vi "MSGR subVI_template 2.vi"(8 "error in (no error)":errorcluster, 11 "MSGR Q name":T1) -> (0 "error out":errorcluster)   [LabVIEW 2018]
uses:
  MSGR Q Name TypeDef.ctl
  MSGR Send (Name).vi
  MSGR Get Q.vi
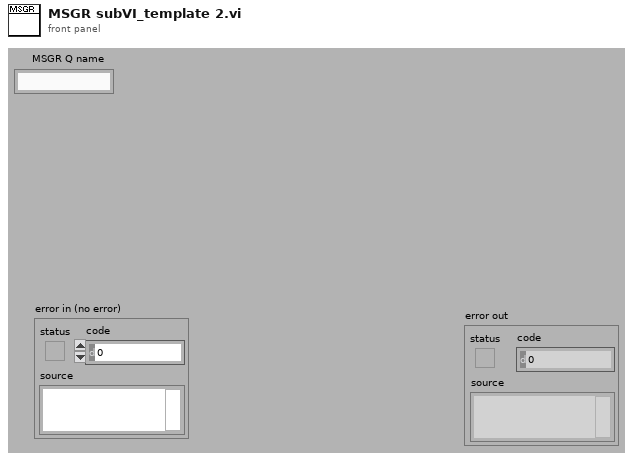
[diagram p1: front panel]
types:
  T1 = typedef "MSGR Q Name TypeDef.ctl" = string
  T2 = typedef "MSGR Q Data TypeDef.ctl" = cluster{"Msg":string, "Parameters":string, "Reply?":bool, "ReplyQ":string}
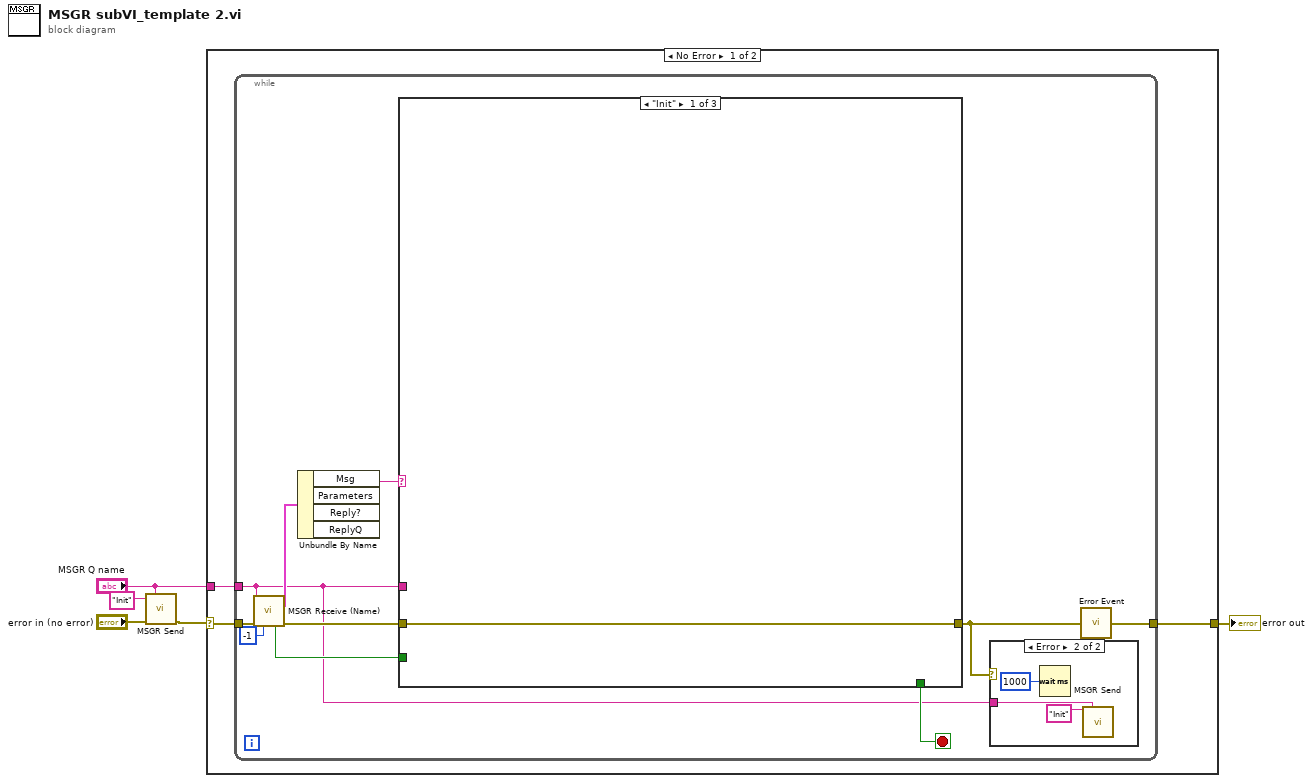
[diagram p0: block diagram]
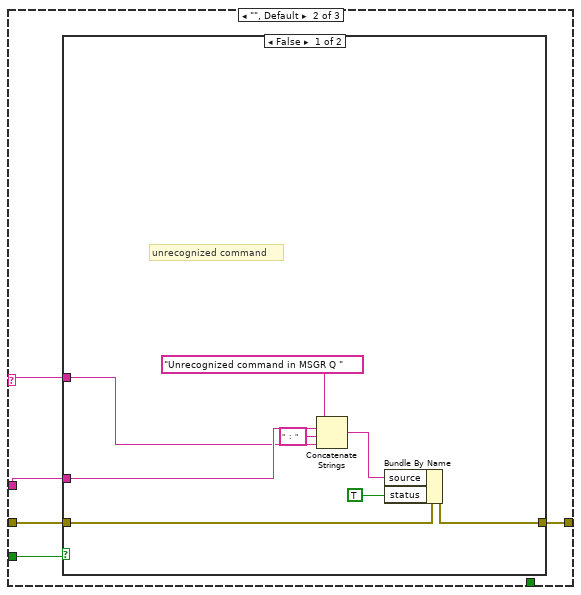
[diagram p3: hidden frame]
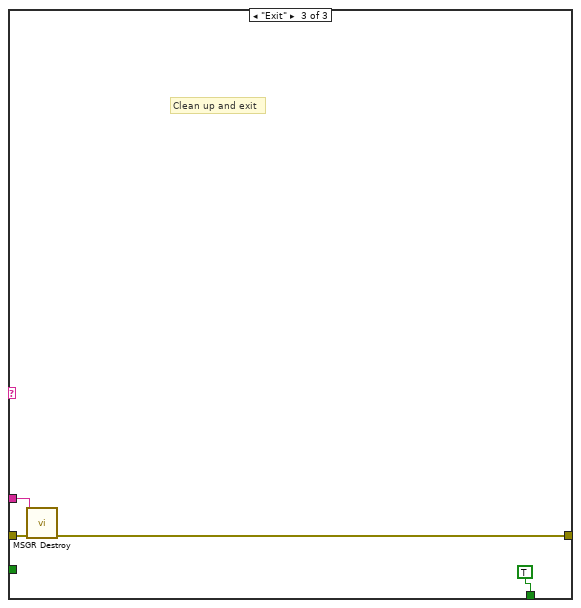
[diagram p5: hidden frame]
diagram:
  n1 = call-poly "MSGR Send.vi"("Msg"="Init", "MSGR Q name"="MSGR Q name", "error in (no error)"="error in (no error)") -> ("error out"=w4:errorcluster)  [unwired: 11 in, 1 out]
  n2 = case shown="No Error" w4 {
    selector: w4 -> [w8 w41]
    tunnel: [w7 w41] -> w5
    tunnel: "MSGR Q name" -> [w6 _]
    frame No Error {
      n3 = while {
        tunnel: w8 -> [w18]
        tunnel: [w11] -> w7
        tunnel: w6 -> [w9]
        stop <- w14 stop-if-true
        n4 = call "MSGR Receive (Name).vi"("MSGR Q name"=w9, "error in (no error)"=w18, "timeout in ms (-1)"=-1) -> ("MSGR Q Data TypeDef"=w16:T2, "timed out?"=w13:bool, "error out"=w17:errorcluster)  [unwired: 10 out]
        n5 = Unbundle By Name(w16) -> ("Msg"=w15:string)  [unwired: 3 out]
        n6 = case shown="\"Init\"" w15 {
          selector: w15 -> [_ w24 _]
          tunnel: w17 -> [w22 w27 w40]
          tunnel: [w22 w26 w38] -> w10
          tunnel: [_ _ TRUE] -> w14
          tunnel: w9 -> [_ w25 w37]
          tunnel: w13 -> [_ w23 _]
          frame "Init" {
          }
          frame "", Default {
            n7 = case shown="False" w23 {
              tunnel: w27 -> [w35 w36]
              tunnel: [w34 w36] -> w26
              tunnel: w25 -> [w30 _]
              tunnel: w24 -> [w28 _]
              frame False {
                # "unrecognized command"
                n8 = Concatenate Strings("Unrecognized command in MSGR Q " ("source"), w30, "  :  " ("string"), w28) -> (w31:string)
                n9 = Bundle By Name(cluster=w35, "source"=w31, "status"=TRUE) -> (w34:errorcluster)
              }
              frame True {
                # "default time out action"
              }
            }
          }
          frame "Exit" {
            # "Clean up and exit"
            n10 = call "MSGR Destroy.vi"("MSGR Q name"=w37, "error in (no error)"=w40) -> ("error out"=w38:errorcluster)  [unwired: 13 out]
          }
        }
        n11 = case shown="Error" w10 {
          tunnel: w9 -> [_ w19]
          frame No Error {
          }
          frame Error {
            n12 = Wait (ms)(milliseconds to wait=u32 1000) -> ()  [unwired: 1 out]
            n13 = call-poly "MSGR Send.vi"("Msg"="Init", "MSGR Q name"=w19) -> ()  [unwired: 12 in, 2 out]
          }
        }
        n14 = call "Error Event.vi"("error in (no error)"=w10) -> ("error out"=w11:errorcluster)  [unwired: 1 in, 5 out]
      }
    }
    frame Error {
    }
  }
  "error out" <- w5
